vi "_Open_Port.vi"(8 "error in (no error)":errorcluster, 11 "Postgres Connector.lvclass":refnum<class "Postgres Connector.lvclass">) -> (0 "error out":errorcluster, 3 "output cluster":refnum<class "Postgres Connector.lvclass">)   [LabVIEW 2020, in "Postgres Connector.lvclass"]
doc: "Establish a TCP connection with the server where the database is installed."
uses:
  Postgres Connector.lvclass
  Postgres Connector.lvclass/Postgres Connector.ctl
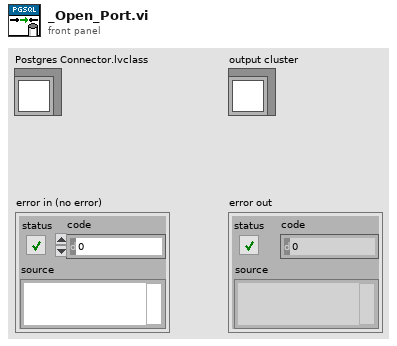
[diagram p1: front panel]
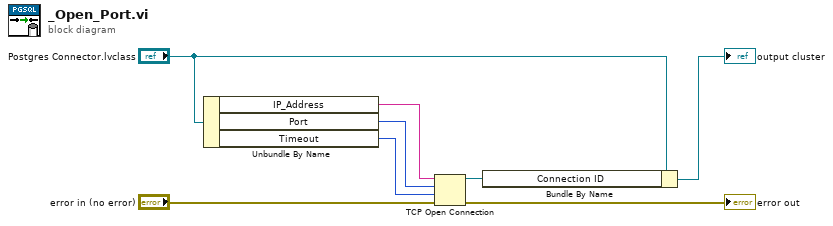
[diagram p0: block diagram]
diagram:
  n1 = Unbundle By Name("Postgres Connector.lvclass") -> ("IP_Address"=w3:string, "Port"=w4:u16, "Timeout"=w2:i32)
  n2 = TCP Open Connection(address=w3, remote port or service name=w4, timeout ms (60000)=w2, error in (no error)="error in (no error)") -> (connection ID=w1:refnum<k5>, error out=→"error out":errorcluster)  [unwired: 1 in]
  n3 = Bundle By Name(cluster="Postgres Connector.lvclass", "Connection ID"=w1) -> (→"output cluster":refnum<class "Postgres Connector.lvclass">)
